vi "GFITS_DBSCollectHeaders.vi"(2 "Database RefNum in":T1, 7 "Keywords":string[][](array[string]), 9 "numer of keywords":i32, 11 "error in (no error)":errorcluster) -> (15 "error out":errorcluster)   [LabVIEW 2016]
uses:
  GFITS_datatypesctl.ctl
  DBSHAND/private/vis/DatabaseHand_RefNum.ctl
panel:
  in  "Types":T2={"TBIT"=1, "TBYTE"=11, "TSTRING"=16, "TSHORT"=21, "TLONG"=41, "TFLOAT"=42, "TDOUBLE"=82, "TCOMPLEX"=83, "TDBLCOMPLEX"=163, "TUINT"=30, "TUSHORT"=20, "TULONG"=40, "TINT"=31, "TSBYTE"=12, "TLONGLONG"=81, "TLOGICAL"=14}
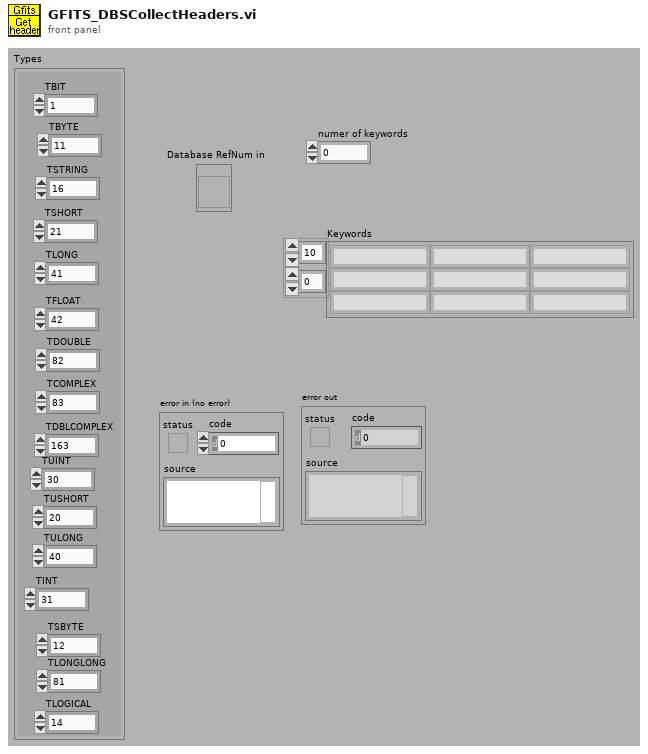
[diagram p1: front panel]
types:
  T1 = typedef "DatabaseHand_RefNum.ctl" = refnum<vi>
  T2 = typedef "GFITS_datatypesctl.ctl" = cluster{"TBIT":i32, "TBYTE":i32, "TSTRING":i32, "TSHORT":i32, "TLONG":i32, "TFLOAT":i32, "TDOUBLE":i32, "TCOMPLEX":i32, "TDBLCOMPLEX":i32, "TUINT":i32, "TUSHORT":i32, "TULONG":i32, "TINT":i32, "TSBYTE":i32, "TLONGLONG":i32, "TLOGICAL":i32}
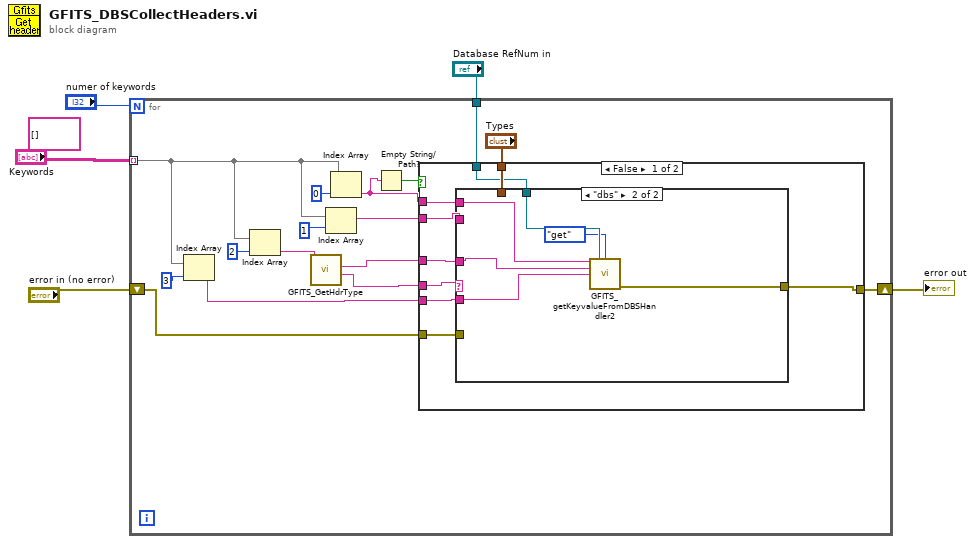
[diagram p0: block diagram]
diagram:
  (unwired) string[][] []
  n1 = for {
    N: "numer of keywords" -> [_]
    tunnel: "Keywords" -> [w16] mode=indexing
    shift-right: [w6] -> w3
    shift-left: "error in (no error)" -> [w11]
    tunnel: "Database RefNum in" -> [w10]
    n2 = Index Array(array=w16, index=3 ("Array Index")) -> (element=w17:string)
    n3 = Index Array(array=w16, index=2 ("Array Index")) -> (element=w9:string)
    n4 = call "GFITS_GetHdrType.vi"("keyval"=w9) -> ("type"=w8:string, "keyval out"=w7:string)  [unwired: 9 out]
    n5 = Index Array(array=w16, index=1 ("Array Index")) -> (element=w18:string)
    n6 = Index Array(array=w16, index=0 ("Index")) -> (element=w14:string)
    n7 = Empty String/Path?(string/path=w14) -> (empty?=w13:bool)
    n8 = case shown="False" w13 {
      tunnel: w18 -> [w29 _]
      tunnel: w17 -> [w26 _]
      tunnel: w8 -> [w27 _]
      tunnel: w7 -> [w28 _]
      tunnel: w14 -> [w30 _]
      tunnel: "Types" -> [w25 _]
      tunnel: [w23 w38] -> w6
      tunnel: w11 -> [w22 w38]
      tunnel: w10 -> [w24 _]
      frame False {
        n9 = case shown="\"dbs\"" w27 {
          tunnel: w26 -> [_ w34]
          tunnel: w29 -> [_ _]
          tunnel: w28 -> [_ w35]
          tunnel: w30 -> [_ w36]
          tunnel: w25 -> [_ _]
          tunnel: w24 -> [_ w37]
          tunnel: [w31 w32] -> w23
          tunnel: w22 -> [w31 _]
          frame Default {
          }
          frame "dbs" {
            n10 = call "GFITS_getKeyvalueFromDBSHandler2.vi"("key name in header"=w36, "Database RefNum in"=w37, "action"=enum16{"get", "clear"}."get", "varname"=w35, "comment"=w34) -> ("error out"=w32:errorcluster)  [unwired: 4 in, 6 out]
          }
        }
      }
      frame True {
      }
    }
  }
  "error out" <- w3
